vi "Задание_АБ_система.vi"() -> ()   [LabVIEW 2017]
uses:
  <vilib>/Analysis/baseanly.llb/Mean (DBL).vi
  <vilib>/gmath/statdist.llb/Normal Random.vi
  <vilib>/Analysis/3filter.llb/Bessel Filter (DBL).vi
  <vilib>/Analysis/NI_AALBase.lvlib
  <vilib>/gmath/NI_Gmath.lvlib
panel:
  out "x*y 2":i32
  out "x*y":i32
  out "size(s) 2":i32[](array[numeric])
  out "Размер окна с паузами":i32
  out "size(s)":i32
  out "output array":dbl[](array[numeric])
  out "Декодированное сообщение":dbl[](array[numeric])
  in  "Кол-во копий":i32=5
  out "Подготовленный к отправке мажоритарный код":dbl[][](array[numeric])
  out "Демодулированный сигнал 2":i16[](graph)
  out "0, 1":i16[](array[numeric])
  in  "Пороговое значение 2":dbl
  out "Среднее значение":dbl[](array[numeric])
  out "Шум на основе распределения Рэлея":dbl[](graph)
  out "Демодулированный и отфильтрованный сигнал":dbl[](graph)
  in  "Нижняя частота среза":dbl
  in  "Порядок фильтра":i64(slide) scale=0.0..20.0
  in  "Переменная floor(x/y)":i32
  out "Модулирующий сигнал":dbl[](graph)
  out "Частотно модулированный цифровой сигнал":dbl[](graph)
  in  "см. 1.2 Циклов в секунду":i32(slide) scale=4.0..50.0
  in  "Сколько битов брать":i32=4
  out "Радио сигнал с паузами":dbl[](graph)
  in  "Кол-во выборок":i32=400
  out "Массив с паузами":dbl[](array[numeric])
  in  "Количество бит":i32=8
  out "Вырезка из массива":dbl[](array[numeric])
  out "Биты на выходе 1":dbl[](array[numeric])
  # "Демодуляция"
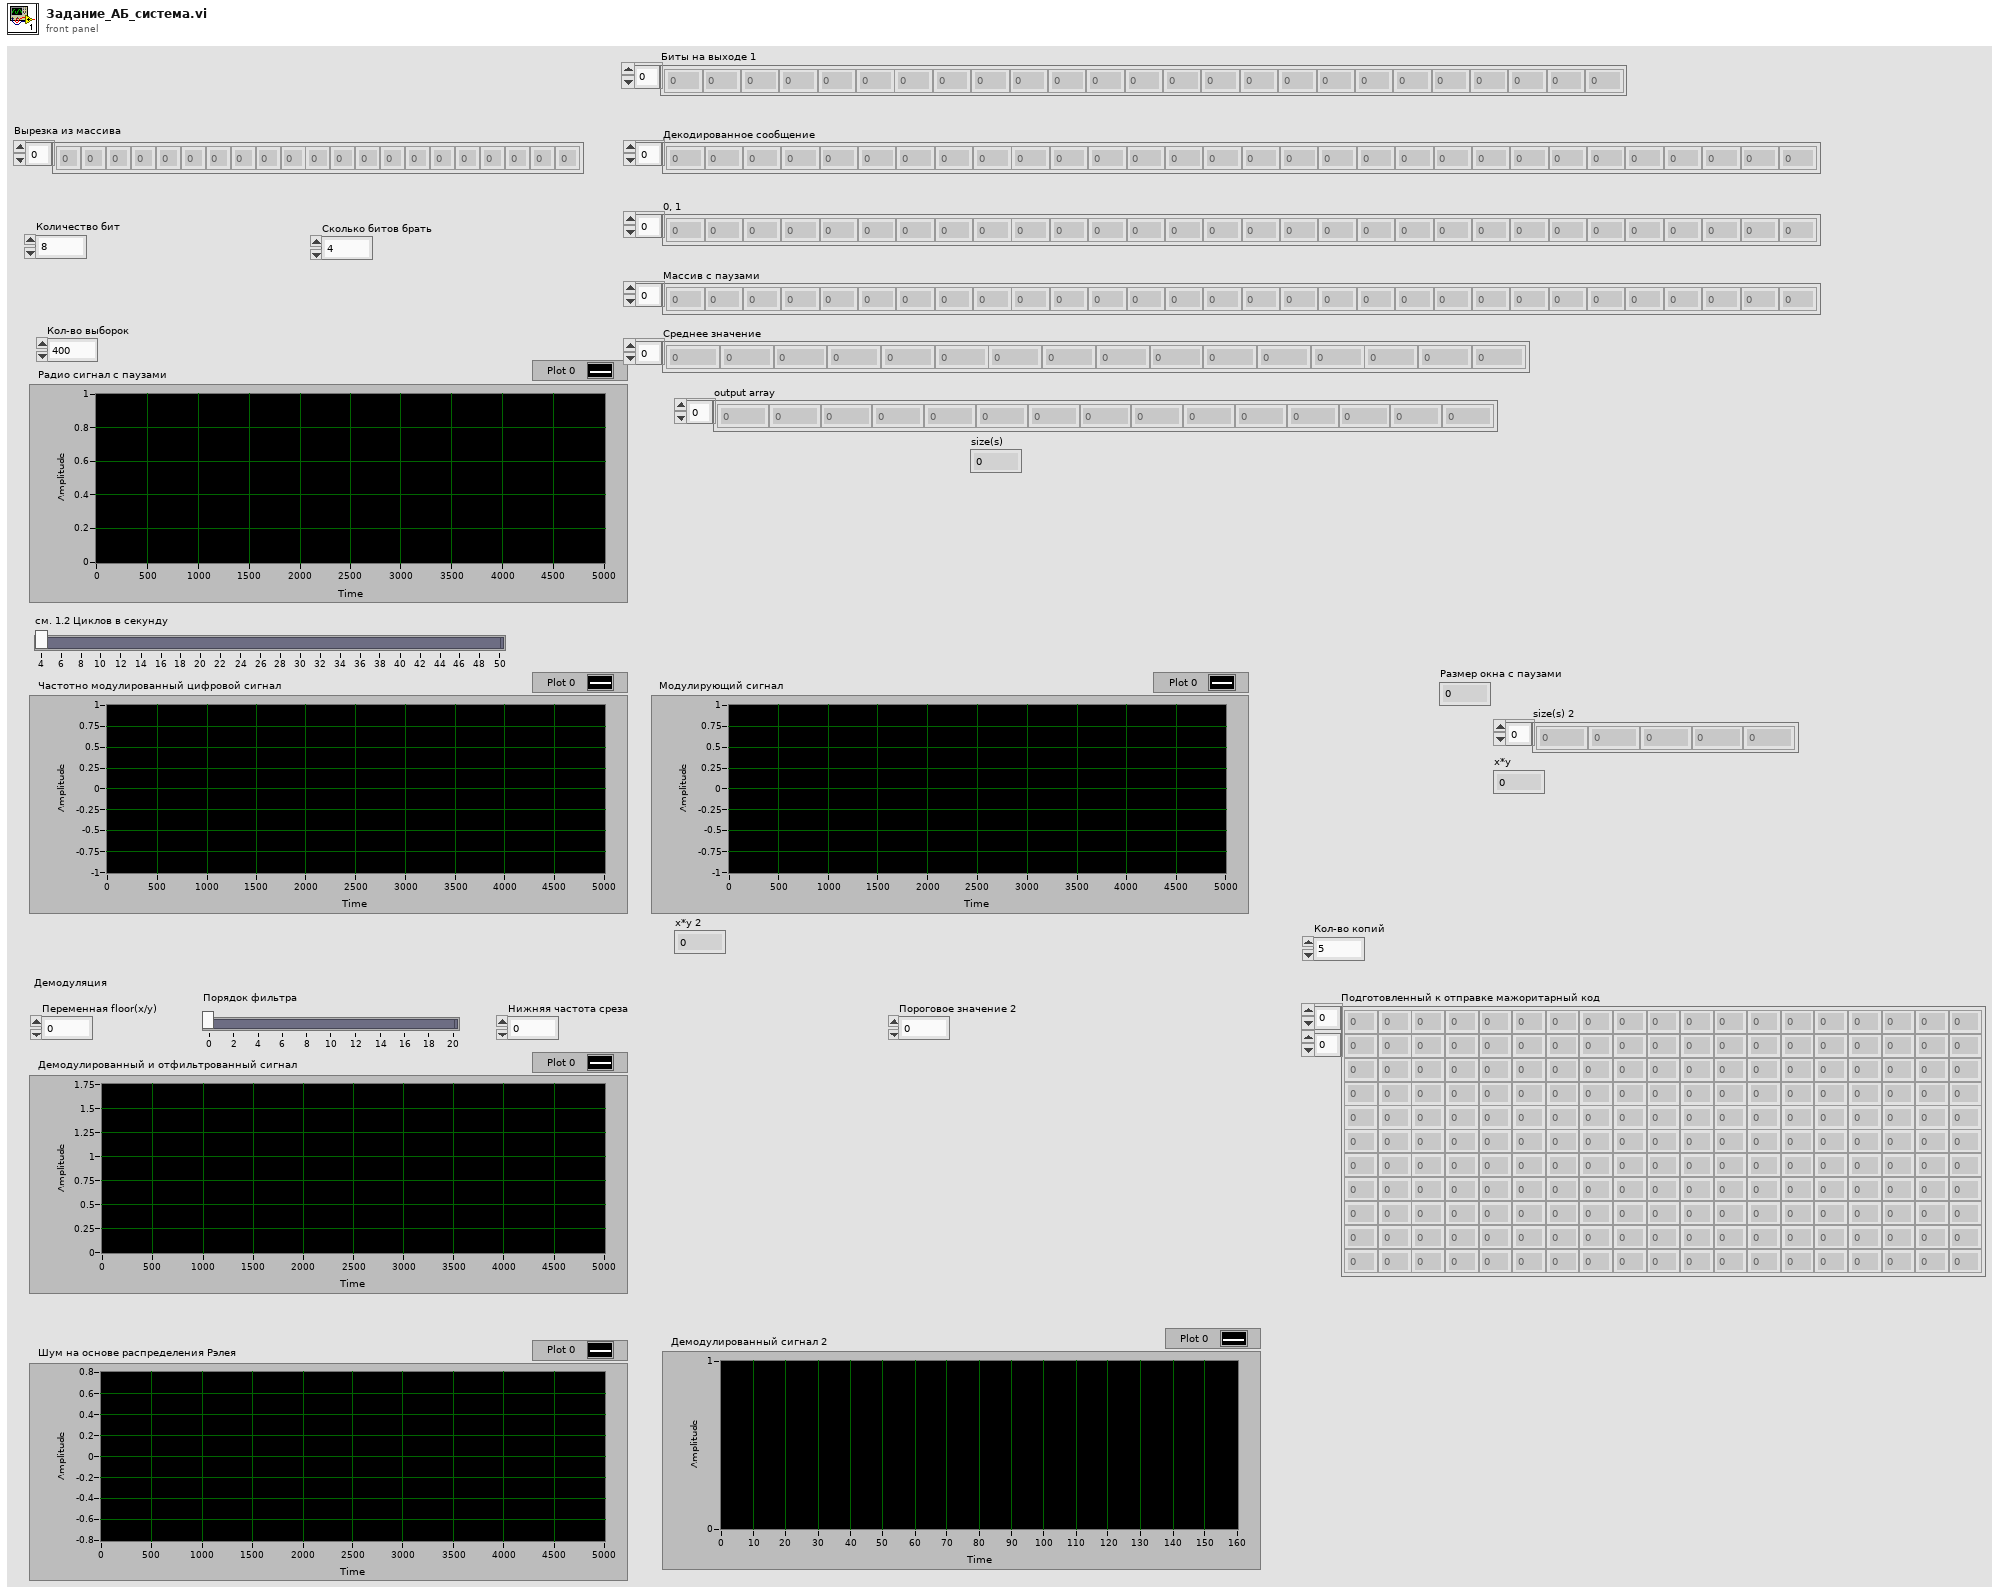
[diagram p1: front panel]
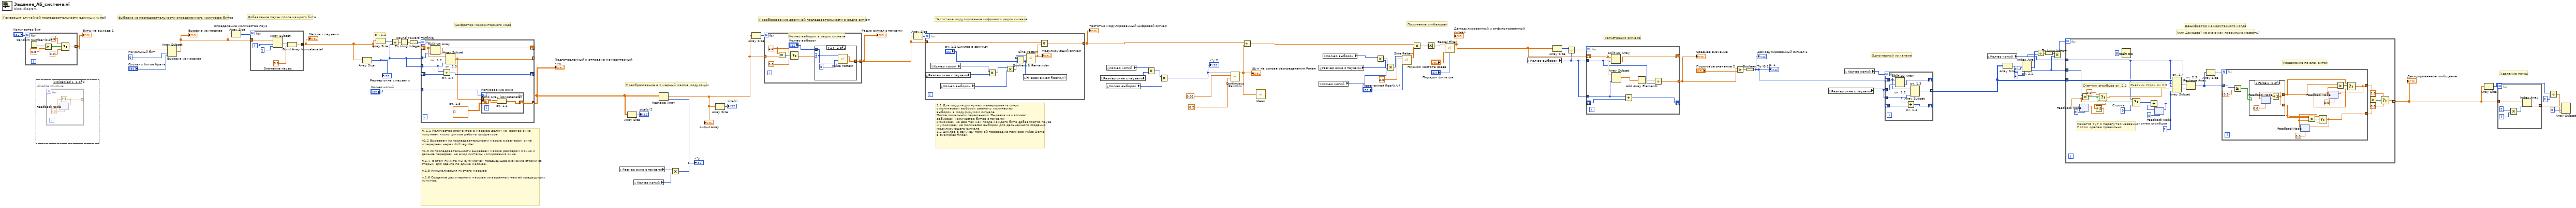
[diagram p0: block diagram]
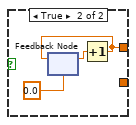
[diagram p3: hidden frame]
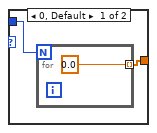
[diagram p4: hidden frame]
diagram:
  w70 = 0  # Начальный бит
  # "Удаление паузы"
  # "(или Декодер? не знаю как правильно назвать)"
  # "Дешифратор мажоритарного когда"
  # "Одномерный из канала"
  # "Получение огибающей"
  # "Регистрация сигнала"
  # "Преобразование в 1 мерный массив модуляции"
  # "п. 1.1 Количество элементов в массиве делим на  размер окна\nполучаем число циклов работы шифратора\n\nп1.2 Вырезаем из последовательности массив с размером окна \nи передаем через shift register\n\nп1.3 Из последовательности вырезаем массив размером с окно и \nдальше передаем на вход системы копирования окна.\n \nп.1.4  В этом пункте мы суммируем предыдущее значение строки со\nстарым для сдвига по длине массива.\n\nп.1.5 Инициализация пустого массива\n\nп.1.6 Создание двухмерного массива из выранных частей предыдущих\nпунктов."
  # "см. 1.1"
  # "Шифратор мажоритарного кода"
  # "1.1 Для модуляции нужно сгенерировать синус \nс количесвом выборок равному количеству \nвыборок в модулирумом сигнале\nПосле локальной переменной !Вырезка из массива! \nЗабираем количество битов с паузами \nУмножаем на два так как после каждого бита добавляется пауза\nи умножаем на Количесво выборок для дальнейшого создания  \nмодулирующего сигнала\n1.2 Циклов в секунду прямой перевод из примера Pulse Demo \nв Examples Finder."
  # "Преобразование двоичной последовательности в радио сигнал"
  # "Частотное модулирование цифрового радио сигнала"
  # "Добавление паузы после каждого бита"
  # "Выборка из последовательности определенного количесва битов"
  # "Генерация случайной последовательности единиц и нулей"
  n1 = for {
    N: "Количество бит" -> [_]
    tunnel: [w72] -> w68 mode=indexing
    n2 = Random Number (0-1)() -> (number: 0 to 1=w77:dbl)
    n3 = Greater Or Equal?(x=w77, y=0.5) -> (x >= y?=w75:bool)
    n4 = Select(t=1.0, s=w75, f=0.0) -> (s? t:f=w72:dbl)
  }
  "Биты на выходе 1" <- w68
  n5 = disable-structure shown="Disabled" {
    frame Disabled {
      n6 = for {
        tunnel: [w78] -> _ mode=indexing
        n7 = feedback #1(0.0) -> (w80:dbl)
        n8 = Increment(x=w80) -> (x+1=w78:dbl)
        n9 = feedback-in #1(w78) -> ()
      }
    }
    frame Enabled {
    }
  }
  n10 = Array Subset "Вырезка из массива"(array=w68, index=w70, length="Сколько битов брать") -> (w66:dbl[])
  "Вырезка из массива" <- w66
  n11 = Array Size "Определение количества пауз"(array=w66) -> (size(s)=w67:i32)
  n12 = for {
    N: w67 -> [_]
    tunnel: w66 -> [w83]
    tunnel: [w82] -> w18 mode=concatenating
    i -> [w81]
    w84 = 0.0  # Значение паузы
    n13 = Array Subset(array=w83, index=w81, length=1) -> (w85:dbl[])
    n14 = Build Array (concatenate)(w85, w84) -> (w82:dbl[])
  }
  "Массив с паузами" <- w18
  n15 = Array Size(array=w18) -> (size(s)=w17:i32)
  "Размер окна с паузами" <- w17
  n16 = Array Size(array=w18) -> (size(s)=w40:i32)
  n17 = Divide(x=w40, y=w17) -> (x/y=w39:dbl)
  n18 = Round Toward +Infinity(x=w39) -> (ceil(x): smallest int >= x=w38:dbl)
  n19 = To Long Integer(number=w38) -> (32bit integer=w37:i32)
  n20 = for {
    N: w37 -> [_]
    shift-right: [w96] -> _
    shift-left: w18 -> [w94]
    tunnel: w17 -> [w95]
    shift-right: [w92] -> _
    shift-left: _ -> [w91]
    tunnel: w17 -> [w93]
    tunnel: [w90] -> _ mode=indexing
    tunnel: [w89] -> w16 mode=concatenating
    tunnel: "Кол-во копий" -> [w87]
    w88 = dbl[][] []  # см. 1.5
    n21 = Split 1D Array "см. 1.2"(array=w94, index=w95) -> (second subarray=w96:dbl[])  [unwired: 1 out]
    n22 = Add "см. 1.4"(x=w93, y=w91) -> (x+y=w92:i32)
    n23 = Array Subset "см. 1.3"(array=w94, length=w93) -> (w90:dbl[])  [unwired: 1 in]
    n24 = for "Копирование окна" {
      N: w87 -> [_]
      tunnel: w90 -> [w98]
      shift-right: [w99] -> w89
      shift-left: w88 -> [w97]
      n25 = Build Array (concatenate) "см. 1.6"(w97, w98) -> (w99:dbl[][])
    }
  }
  "Подготовленный к отправке мажоритарный код" <- w16
  n26 = local read "Размер окна с паузами"() -> (w35:i32)
  n27 = Array Size(array=w16) -> (size(s)=→"size(s) 2":i32[])
  n28 = local read "Кол-во копий"() -> (w34:i32)
  n29 = Multiply(x=w35, y=w34) -> (x*y=w33:i32)
  "x*y" <- w33
  n30 = Reshape Array(w16, w33) -> (w20:dbl[])
  "output array" <- w20
  n31 = Array Size(array=w20) -> (size(s)=→"size(s)":i32)
  n32 = Array Size(array=w20) -> (size(s)=w64:i32)
  n33 = for {
    N: w64 -> [_]
    tunnel: [w102] -> w63 mode=concatenating
    tunnel: w20 -> [w100] mode=indexing
    w105 = 1.0
    # "Кол-во выборок в радио сигнале"
    n34 = Equal?(x=w105, y=w100) -> (x = y?=w106:bool)
    n35 = Select(t=w105, s=w106, f=0.0) -> (s? t:f=w103:dbl)
    n36 = case shown="1" w103 {
      tunnel: [w107 w111] -> w102
      tunnel: "Кол-во выборок" -> [w108 w110]
      frame 0, Default {
        n37 = for {
          N: w108 -> [_]
          tunnel: [0.0] -> w107 mode=indexing
        }
      }
      frame 1 {
        n38 = call <vilib>:"Pulse Pattern.vi"("width"=w110, "delay"=0, "samples"=w110) -> ("Pulse Pattern"=w111:dbl[])  [unwired: 1 in, 1 out]
      }
    }
  }
  "Радио сигнал с паузами" <- w63
  n39 = Array Size(array=w63) -> (size(s)=w65:i32)
  n40 = for {
    N: w65 -> [_]
    tunnel: w63 -> [w121]
    tunnel: [w120] -> w48
    n41 = local read "Размер окна с паузами"() -> (w115:i32)
    n42 = local read "Кол-во копий"() -> (w114:i32)
    n43 = local read "Кол-во выборок"() -> (w118:i32)
    n44 = Multiply(x=w114, y=w115) -> (x*y=w113:i32)
    n45 = Multiply(x=w113, y=w118) -> (x*y=w117:i32)
    n46 = Quotient & Remainder(x=w117, y="см. 1.2 Циклов в секунду") -> (floor(x/y)=w116:i32)  [unwired: 1 out]
    n47 = local write "Переменная floor(x/y)"(w116) -> ()
    n48 = call <vilib>:"Sine Pattern.vi"("cycles"=w116, "samples"=w117) -> ("Sinusoidal Pattern"=w119:dbl[])  [unwired: 2 in, 1 out]
    "Модулирующий сигнал" <- w119
    n49 = Multiply(x=w121, y=w119) -> (x*y=w120:dbl[])
  }
  "Частотно модулированный цифровой сигнал" <- w48
  n50 = local read "Размер окна с паузами"() -> (w50:i32)
  n51 = local read "Кол-во выборок"() -> (w12:i32)
  n52 = local read "Кол-во копий"() -> (w51:i32)
  n53 = Multiply(x=w51, y=w50) -> (x*y=w14:i32)
  n54 = Multiply(x=w14, y=w12) -> (x*y=w13:i32)
  "x*y 2" <- w13
  n55 = call-poly <vilib>:"Continuous Random.vi"("std"=0.2 ("b"), "mean"=0.01 ("x"), "samples"=w13) -> ("normal random data"=w49:dbl[])  [unwired: 7 in, 1 out]
  "Шум на основе распределения Рэлея" <- w49
  n56 = Add(x=w48, y=w49) -> (x+y=w47:dbl[])
  n57 = call-poly <vilib>:"Mean.vi"("X"=w49) -> ()  [unwired: 2 out]
  n58 = local read "Размер окна с паузами"() -> (w54:i32)
  n59 = local read "Кол-во копий"() -> (w9:i32)
  n60 = local read "Кол-во выборок"() -> (w55:i32)
  n61 = Multiply(x=w55, y=w54) -> (x*y=w11:i32)
  n62 = Multiply(x=w11, y=w9) -> (x*y=w10:i32)
  n63 = call <vilib>:"Sine Pattern.vi"("cycles"="Переменная floor(x/y)", "amplitude"=2.0, "samples"=w10) -> ("Sinusoidal Pattern"=w56:dbl[])  [unwired: 1 in, 1 out]
  n64 = Multiply(x=w47, y=w56) -> (x*y=w60:dbl[])
  n65 = Absolute Value(x=w60) -> (abs(x)=w57:dbl[])
  n66 = call-poly <vilib>:"Bessel Filter.vi"("order"="Порядок фильтра", "low cutoff freq: fl"="Нижняя частота среза", "X"=w57) -> ("Filtered X"=w45:dbl[])  [unwired: 5 in, 1 out]
  "Демодулированный и отфильтрованный сигнал" <- w45
  n67 = local read "Кол-во выборок"() -> (w44:i32)
  n68 = Array Size(array=w45) -> (size(s)=w46:i32)
  n69 = Divide(x=w46, y=w44) -> (x/y=w21:dbl)
  n70 = for {
    N: w21 -> [_]
    tunnel: w44 -> [w124]
    shift-right: [w131] -> _
    shift-left: w45 -> [w130]
    tunnel: w44 -> [w127]
    shift-right: [w128] -> _
    shift-left: _ -> [w129]
    tunnel: [w123] -> w42 mode=indexing
    n71 = Split 1D Array(array=w130, index=w124) -> (second subarray=w131:dbl[])  [unwired: 1 out]
    n72 = Array Subset(array=w130, length=w127) -> (w126:dbl[])  [unwired: 1 in]
    n73 = Add(x=w127, y=w129) -> (x+y=w128:i32)
    n74 = Add Array Elements(numeric array=w126) -> (sum=w125:dbl)
    n75 = Divide(x=w125, y=w124) -> (x/y=w123:dbl)
  }
  "Среднее значение" <- w42
  n76 = Greater?(x=w42, y="Пороговое значение 2") -> (0:w41:bool[])
  n77 = Boolean To (0,1)(Boolean=w41) -> (0, 1=w23:i16[])
  "0, 1" <- w23
  "Демодулированный сигнал 2" <- w23
  n78 = local read "Размер окна с паузами"() -> (w22:i32)
  n79 = local read "Кол-во копий"() -> (w8:i32)
  n80 = for {
    N: w8 -> [_]
    shift-right: [w138] -> _
    shift-left: w23 -> [w136]
    tunnel: w22 -> [w137]
    shift-right: [w134] -> _
    shift-left: _ -> [w133]
    tunnel: w22 -> [w135]
    tunnel: [w132] -> w24 mode=indexing
    n81 = Split 1D Array "см. 1.2"(array=w136, index=w137) -> (second subarray=w138:i16[])  [unwired: 1 out]
    n82 = Add "см. 1.4"(x=w135, y=w133) -> (x+y=w134:i32)
    n83 = Array Subset "см. 1.3"(array=w136, length=w135) -> (w132:i16[])  [unwired: 1 in]
  }
  n84 = local read "Кол-во копий"() -> (w25:i32)
  n85 = Array Size(array=w24) -> (size(s)=w32:i32[])
  n86 = Index Array "см. 2.1"(array=w32, index #1=0 ("index"), index #2=1 ("index")) -> (element #1=w29:i32, element #2=w28:i32)
  n87 = Divide(x=w29, y=w25) -> (x/y=w27:dbl)
  n88 = To Long Integer(number=w27) -> (32bit integer=w26:i32)
  n89 = Multiply(x=w26, y=w28) -> (x*y=w7:i32)
  n90 = for {
    N: w7 -> [_]
    tunnel: w24 -> [w162]
    tunnel: w28 -> [w154]
    tunnel: w25 -> [w147]
    tunnel: [w141] -> w1 mode=indexing
    w161 = 1  # кол-во столбцов
    w152 = 0  # Строка
    # "Разделение по элементам"
    # "Кажется тут я перепутал названия  \nПотом сделаю правильно"
    # "Счетчик строк см 2.3"
    # "Счетчик столбцов см. 2.2"
    n91 = feedback #2(0) -> (w150:dbl)
    n92 = Equal?(x=w154, y=w150) -> (x = y?=w156:bool)
    n93 = Select(t=0.0, s=w156, f=w150) -> (s? t:f=w149:dbl)
    n94 = Increment(x=w149) -> (x+1=w148:dbl)
    n95 = feedback-in #2(w148) -> ()
    n96 = Wait (ms)(milliseconds to wait=u32 0) -> ()  [unwired: 1 out]
    n97 = Select(t=w147, s=w156, f=w152) -> (s? t:f=w153:i32)
    n98 = feedback #3(0) -> (w155:i32)
    n99 = Add(x=w153, y=w155) -> (x+y=w151:i32)
    n100 = feedback-in #3(w151) -> ()
    n101 = Array Subset "см. 2.4"(array=w162, index (row)=w151, length (row)=w147, index (col)=w149, length (col)=w161) -> (w163:i16[][])
    n102 = Reshape Array "см. 2.5"(w163, w147) -> (w145:i16[])
    n103 = Array Size(array=w145) -> (size(s)=w146:i32)
    n104 = for {
      N: w146 -> [_]
      tunnel: w145 -> [w174] mode=indexing
      tunnel: [w169] -> w140
      tunnel: [w165] -> w139
      n105 = Greater Or Equal?(x=w174, y=0.5) -> (x >= y?=w175:bool)
      n106 = case shown="False" w175 {
        tunnel: [_ w180] -> w173
        tunnel: [w177 _] -> w172
        frame False {
          n107 = feedback #4(0.0) -> (w178:dbl)
          n108 = Increment(x=w178) -> (x+1=w177:dbl)
          n109 = feedback-in #4(w177) -> ()
        }
        frame True {
          n110 = feedback #5(0.0) -> (w181:dbl)
          n111 = Increment(x=w181) -> (x+1=w180:dbl)
          n112 = feedback-in #5(w180) -> ()
        }
      }
      n113 = feedback #6(0.0) -> (w164:dbl)
      n114 = Greater?(x=w172, y=w164) -> (0:w171:bool)
      n115 = Select(t=w172, s=w171, f=w164) -> (s? t:f=w169:dbl)
      n116 = feedback-in #6(w169) -> ()
      n117 = feedback #7(0.0) -> (w167:dbl)
      n118 = Greater?(x=w173, y=w167) -> (0:w168:bool)
      n119 = Select(t=w173, s=w168, f=w167) -> (s? t:f=w165:dbl)
      n120 = feedback-in #7(w165) -> ()
    }
    n121 = Greater?(x=w139, y=w140) -> (0:w144:bool)
    n122 = Select(t=1.0, s=w144, f=0.0) -> (s? t:f=w141:dbl)
  }
  "Декодированное сообщение" <- w1
  n123 = Array Size(array=w1) -> (size(s)=w4:i32)
  n124 = for {
    N: w4 -> [_]
    tunnel: w1 -> [w187]
    tunnel: [w184] -> w6 mode=indexing
    i -> [w185]
    n125 = Multiply(x=2, y=w185) -> (x*y=w183:i32)
    n126 = Index Array(array=w187, index=w183) -> (element=w184:dbl)
  }
  n127 = Divide(x=w4, y=2) -> (x/y=w2:dbl)
  n128 = Array Subset(array=w6, index=0, length=w2) -> ()  [unwired: 1 out]
